vi "CheckHand.vi"(8 "error in (no error)":errorcluster, 10 "7_1/7_2":bool, 11 "CardHand in":refnum<class "CardHand.lvclass">) -> (0 "error out":errorcluster, 3 "CardHand out":refnum<class "CardHand.lvclass">)   [LabVIEW 2021, in "2023.lvlib" / "CardHand.lvclass"]
uses:
  CardHand.lvclass
  CardHand.lvclass/CardHand.ctl
  <userlib>/_OpenG.lib/array/array.llb/Search 1D Array (I32)__ogtk.vi
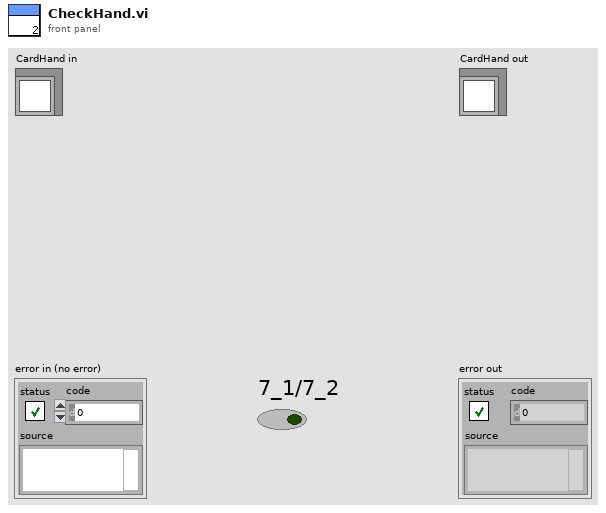
[diagram p1: front panel]
types:
  T1 = enum16{"High Card", "One Pair", "Two Pair", "Three of Kind", "Full House", "Four of Kind", "Five of Kind", "ERROR"}
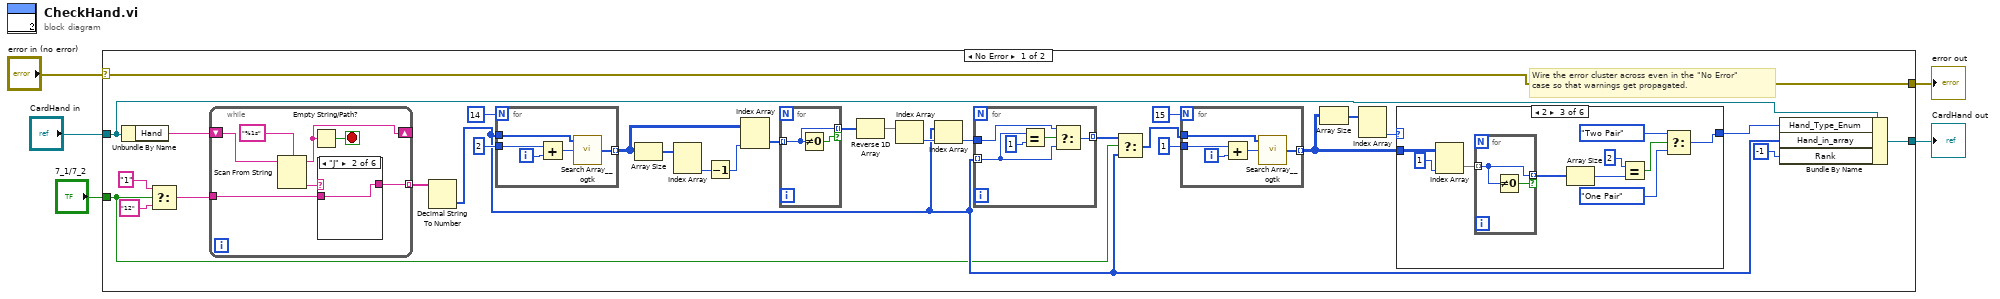
[diagram p0: block diagram]
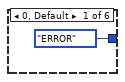
[diagram p2: hidden frame]
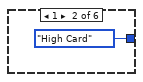
[diagram p3: hidden frame]
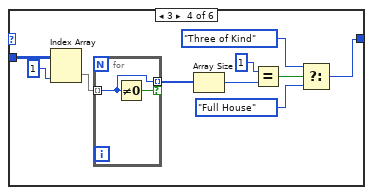
[diagram p4: hidden frame]
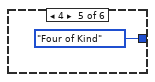
[diagram p5: hidden frame]
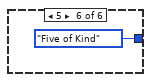
[diagram p6: hidden frame]
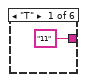
[diagram p7: hidden frame]
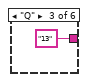
[diagram p8: hidden frame]
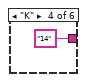
[diagram p9: hidden frame]
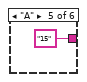
[diagram p10: hidden frame]
diagram:
  n1 = case shown="No Error" "error in (no error)" {
    selector: "error in (no error)" -> [w35 w95]
    tunnel: [w35 w95] -> w4
    tunnel: [w34 w94] -> w3
    tunnel: "CardHand in" -> [w33 w94]
    tunnel: "7_1/7_2" -> [w6 _]
    frame No Error {
      # "Wire the error cluster across even in the \"No Error\"\ncase so that warnings get propagated."
      n2 = Unbundle By Name(w33) -> ("Hand"=w7:string)
      n3 = Select(t="1", s=w6, f="12") -> (s? t:f=w8:string)
      n4 = while {
        shift-right: [w85] -> _
        shift-left: w7 -> [w86]
        tunnel: [w82] -> w32 mode=indexing
        tunnel: w8 -> [w81]
        stop <- w84 stop-if-true
        n5 = Scan From String(format string="%1s", input string=w86) -> (remaining string=w85:string, output 1=w83:string)  [unwired: 3 in, 2 out]
        n6 = Empty String/Path?(string/path=w85) -> (empty?=w84:bool)
        n7 = case shown="\"J\"" w83 {
          selector: w83 -> [_ _ _ _ _ w93]
          tunnel: ["11" w89 "13" "14" "15" w93] -> w82
          tunnel: w81 -> [_ w89 _ _ _ _]
          frame "T" {
          }
          frame "J" {
          }
          frame "Q" {
          }
          frame "K" {
          }
          frame "A" {
          }
          frame Default {
          }
        }
      }
      n8 = Decimal String To Number(string=w32) -> (number=w16:i32[])  [unwired: 2 in, 1 out]
      n9 = for {
        N: 14 -> [_]
        tunnel: w16 -> [w76]
        tunnel: [w80] -> w28 mode=indexing
        tunnel: 2 ("x") -> [w77]
        i -> [w79]
        n10 = Add(x=w77, y=w79) -> (x+y=w78:i32)
        n11 = call-poly <userlib>:"Search Array__ogtk.vi"("Array"=w76, "Element Data"=w78) -> ("Indices of Elements"=w80:i32[])  [unwired: 7 in]
      }
      n12 = Array Size(array=w28) -> (size(s)=w31:i32[])
      n13 = Index Array(array=w31) -> (element #2=w27:i32)  [unwired: 2 in, 1 out]
      n14 = Decrement(x=w27) -> (x-1=w25:i32)
      n15 = Index Array(array=w28, index (col)=w25) -> (element=w26:i32[])  [unwired: 1 in]
      n16 = for {
        tunnel: w26 -> [w75] mode=indexing
        tunnel: [w75] -> w24 mode=indexing if=w74
        n17 = Not Equal To 0?(x=w75) -> (x != 0?=w74:bool)
      }
      n18 = Reverse 1D Array(array=w24) -> (reversed array=w23:i32[])
      n19 = Index Array(array=w23) -> (element=w22:i32)  [unwired: 1 in]
      n20 = Index Array(array=w16, index=w22) -> (element=w21:i32)
      n21 = for {
        tunnel: w16 -> [w70] mode=indexing
        tunnel: w21 -> [w71]
        tunnel: [w69] -> w18 mode=indexing
        n22 = Equal?(x=w70, y=1) -> (x = y?=w72:bool)
        n23 = Select(t=w71, s=w72, f=w70) -> (s? t:f=w69:i32)
      }
      n24 = Select(t=w18, s=w6, f=w16) -> (s? t:f=w17:i32[])
      n25 = for {
        N: 15 -> [_]
        tunnel: w17 -> [w64]
        tunnel: [w68] -> w13 mode=indexing
        tunnel: 1 ("x") -> [w65]
        i -> [w67]
        n26 = Add(x=w65, y=w67) -> (x+y=w66:i32)
        n27 = call-poly <userlib>:"Search Array__ogtk.vi"("Array"=w64, "Element Data"=w66) -> ("Indices of Elements"=w68:i32[])  [unwired: 7 in]
      }
      n28 = Array Size(array=w13) -> (size(s)=w15:i32[])
      n29 = Index Array(array=w15) -> (element #2=w14:i32)  [unwired: 2 in, 1 out]
      n30 = case shown="2" w14 {
        tunnel: [T1."ERROR" ("Hand_Type_Enum") T1."High Card" ("Hand_Type_Enum") w45 w57 T1."Four of Kind" ("Hand_Type_Enum") T1."Five of Kind" ("Hand_Type_Enum")] -> w30
        tunnel: w13 -> [_ _ w47 w59 _ _]
        frame 0, Default {
        }
        frame 1 {
        }
        frame 2 {
          n31 = Index Array(array=w47, index (col)=1 ("disabled index (col)")) -> (element=w39:i32[])  [unwired: 1 in]
          n32 = for {
            tunnel: w39 -> [w49] mode=indexing
            tunnel: [w49] -> w42 mode=indexing if=w48
            n33 = Not Equal To 0?(x=w49) -> (x != 0?=w48:bool)
          }
          n34 = Array Size(array=w42) -> (size(s)=w41:i32)
          n35 = Equal?(x=2, y=w41) -> (x = y?=w38:bool)
          n36 = Select(t=T1."Two Pair" ("Hand_Type_Enum"), s=w38, f=T1."One Pair" ("Hand_Type_Enum")) -> (s? t:f=w45:T1)
        }
        frame 3 {
          n37 = Index Array(array=w59, index (col)=1 ("disabled index (col)")) -> (element=w54:i32[])  [unwired: 1 in]
          n38 = for {
            tunnel: w54 -> [w61] mode=indexing
            tunnel: [w61] -> w53 mode=indexing if=w60
            n39 = Not Equal To 0?(x=w61) -> (x != 0?=w60:bool)
          }
          n40 = Array Size(array=w53) -> (size(s)=w52:i32)
          n41 = Equal?(x=1, y=w52) -> (x = y?=w50:bool)
          n42 = Select(t=T1."Three of Kind" ("Hand_Type_Enum"), s=w50, f=T1."Full House" ("Hand_Type_Enum")) -> (s? t:f=w57:T1)
        }
        frame 4 {
        }
        frame 5 {
        }
      }
      n43 = Bundle By Name(cluster=w33, "Hand_Type_Enum"=w30, "Hand_in_array"=w16, "Rank"=-1) -> (w34:refnum<class "CardHand.lvclass">)
    }
    frame Error {
    }
  }
  "error out" <- w4
  "CardHand out" <- w3
